vi "CheckArmAngle.vi"(9 "Encoder Counts":dbl, 10 "Tolerance  Angle Difference":dbl, 11 "Target Angle":dbl) -> (2 "Positive /Negative":bool, 3 "Outside Tolerance":bool)   [LabVIEW 2013]
doc: "Checks the angle of a motor with a target angle and tolerance angle difference to output a true or false for a positive/ negative movement, and outputs a true or false if it is te range of the outside tolerance."
panel:
  out "Angle Difference":dbl
  # "Positive (true) means raise, negative (false) means lower"
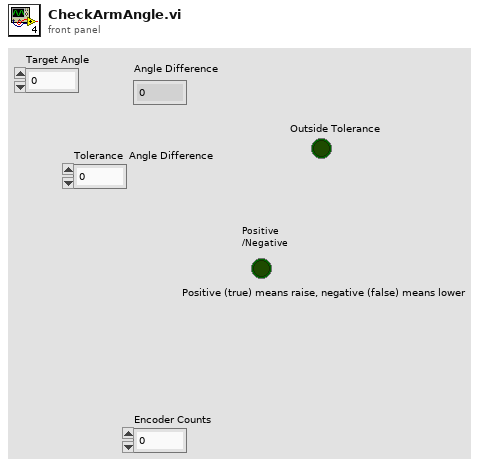
[diagram p1: front panel]
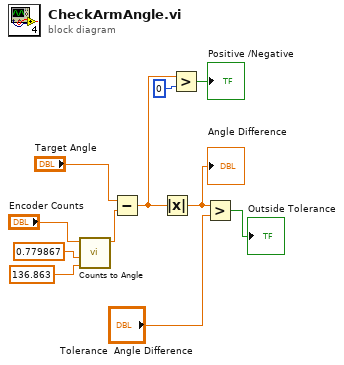
[diagram p0: block diagram]
diagram:
  n1 = call "Counts to Angle.vi"("Slope"=136.863 ("y"), "y-intercept"=0.779867 ("y"), "Input Counts"="Encoder Counts") -> ("Output Angle"=w4:dbl)  [unwired: 8 in]
  n2 = Subtract(x="Target Angle", y=w4) -> (x-y=w7:dbl)
  n3 = Absolute Value(x=w7) -> (abs(x)=w10:dbl)
  "Angle Difference" <- w10
  n4 = Greater?(x=w7, y=0) -> (0:→"Positive /Negative":bool)
  n5 = Greater?(x=w10, y="Tolerance  Angle Difference") -> (0:→"Outside Tolerance":bool)
